vi "Seek Audio File.vi"(8 "error in (no error)":errorcluster, 10 "Frame Position":u64, 11 "Audio File Refnum In":T1) -> (0 "error out":errorcluster, 3 "Audio File Refnum Out":T1)   [LabVIEW 2020, in "G-Audio.lvlib"]
doc: "Seek to the specified frame (sample/ch) in the file being read. Subsequent audio file read will begin at this position. Frame Position is absolute."
uses:
  G-Audio.lvlib
  Controls/Audio File Refnum.ctl
  <vilib>/Utility/error.llb/Error Cluster From Error Code.vi
  lib/g_audio_32.dll
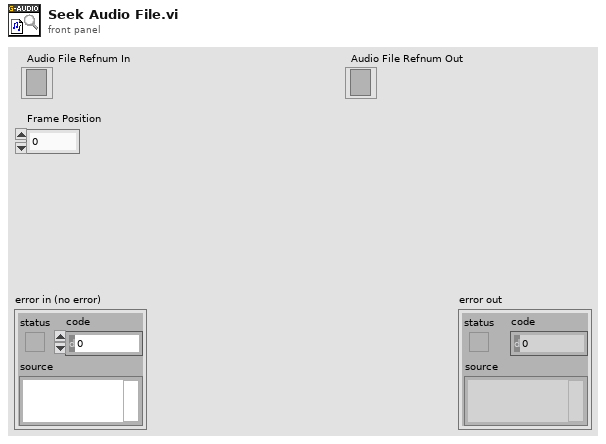
[diagram p1: front panel]
types:
  T1 = typedef "G-Audio.lvlib/Audio File Refnum.ctl" = refnum<file>
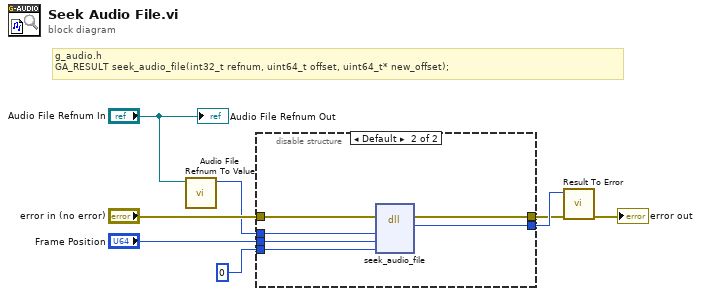
[diagram p0: block diagram]
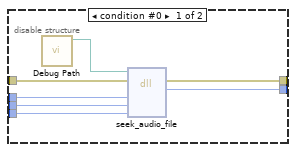
[diagram p2: hidden frame]
diagram:
  # "g_audio.h\nGA_RESULT seek_audio_file(int32_t refnum, uint64_t offset, uint64_t* new_offset);"
  n1 = call "Audio File Refnum To Value.vi"("Audio File Refnum"="Audio File Refnum In") -> ("Refnum Value"=w7:i32)  [unwired: 10 in]
  n2 = disable-structure shown="Default" {
    disable-tunnel: "error in (no error)" -> [w15 w21]
    disable-tunnel: [w13 w19] -> w4
    disable-tunnel: [w14 w20] -> w3
    disable-tunnel: "Frame Position" -> [w12 w18]
    disable-tunnel: w7 -> [w11 w17]
    disable-tunnel: u64 0 -> [w10 w16]
    frame condition #0 {
      n3 = call "Debug Path.vi"() -> ("Debug Path"=w9:path)  [unwired: 11 in]
      n4 = dll-call lib="?" fn="seek_audio_file"(path in=w9, error in=w15, "refnum"=w11, "offset"=w12, "new_offset"=w10) -> (error out=w14:errorcluster, "result"=w13:i32)  [unwired: 4 in, 1 out]
    }
    frame condition #1 (active) {
      n5 = dll-call lib="C:/github/dataflowg/g-audio/src/LabVIEW/G-Audio/lib/g_audio_*.*" fn="seek_audio_file"(error in=w21, "refnum"=w17, "offset"=w18, "new_offset"=w16) -> (error out=w20:errorcluster, "result"=w19:i32)  [unwired: 5 in, 1 out]
    }
  }
  n6 = call "Result To Error.vi"("error in (no error)"=w3, "Result Code"=w4) -> ("error out"=→"error out":errorcluster)  [unwired: 9 in]
  "Audio File Refnum Out" <- "Audio File Refnum In"
